vi "PictureParticleThreshold.vi"(5 "Enum":enum16{"new", "input", "draw", "dump"}(ring), 6 "spotfinding settings":T1={"show all"=FALSE, "threshold/morph"=FALSE, "particle filter"=FALSE, "spot marks"=FALSE, "close filter"=FALSE, "connectivity 4/8"=FALSE, "range"={"Lower value"=30.0, "Upper value"=30.0}, "PSF-size"=0, "Parameters"=[]} {"range"."Upper value" format="%.2f"; "range"."Lower value" format="%.2f"; "Parameters"."Upper Value" format="%.2f"; "Parameters"."Lower Value" format="%.2f"}, 8 "Image Input float":T2, 9 "Image Input 8bit":T2) -> (2 "Image Dst float":T2, 3 "Image Dst 8bit":T2)   [LabVIEW 2009]
uses:
  <vilib>/vision/Image Controls.llb/IMAQ Image.ctl
  spotfindersettings.ctl
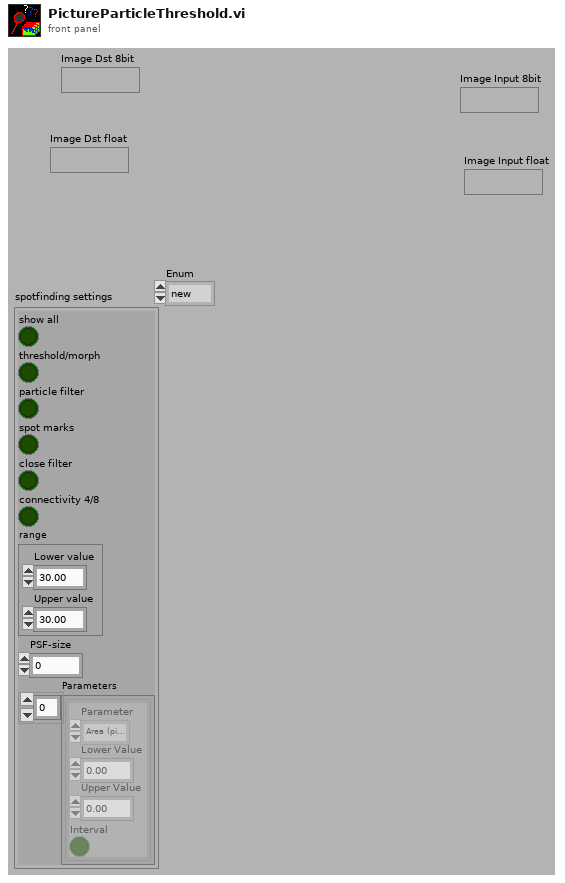
[diagram p1: front panel]
types:
  T1 = typedef "spotfindersettings.ctl" = cluster{"show all":bool, "threshold/morph":bool, "particle filter":bool, "spot marks":bool, "close filter":bool, "connectivity 4/8":bool, "range":cluster{"Lower value":sgl, "Upper value":sgl}, "PSF-size":i32, "Parameters":cluster{"Parameter":enum32{"Area (pixels)", "Area (calibrated)", "Number of holes", "Holes area (pixels)", "Total area (pixels)", "Scanned area (pixels)", "Ratio Area/Scanned area (%)", "Ratio Area/Total area (%)", "Center of mass (X)", "Center of mass (Y)", "Left column (X)", "Upper row (Y)", "Right column (X)", "Lower row (Y)", "Width (pixels)", "Height (pixels)", "Longest segment length", "Longest segment left column (X)", "Longest segment top row  (Y)", "Perimeter", "Holes perimeter", "SumX", "SumY", "SumXX", "SumYY", "SumXY", "Corrected projection X", "Corrected projection Y", "Moment of inertia Ixx", "Moment of inertia Iyy", "Moment of inertia Ixy", "Mean chord X", "Mean chord Y", "Max intercept", "Mean intercept perpendicular", "Particle orientation", "Equivalent ellipse minor axis", "Ellipse major axis", "Ellipse minor axis", "Ratio of equivalent ellipse axis", "Rectangle big side", "Rectangle small side", "Ratio of equivalent rectangle sides", "Elongation factor", "Compactness factor", "Heywood circularity factor", "Type factor", "Hydraulic radius", "Waddel disk diameter", "Diagonal"}, "Lower Value":sgl, "Upper Value":sgl, "Interval":bool}[]}
  T2 = typedef "IMAQ Image.ctl" = refnum<image>
  T3 = enum32{"Gray", "Binary", "Gradient", "Rainbow", "Temperature"}
  T4 = enum16{"Ini", "get", "dump", "set", "draw", "black"}
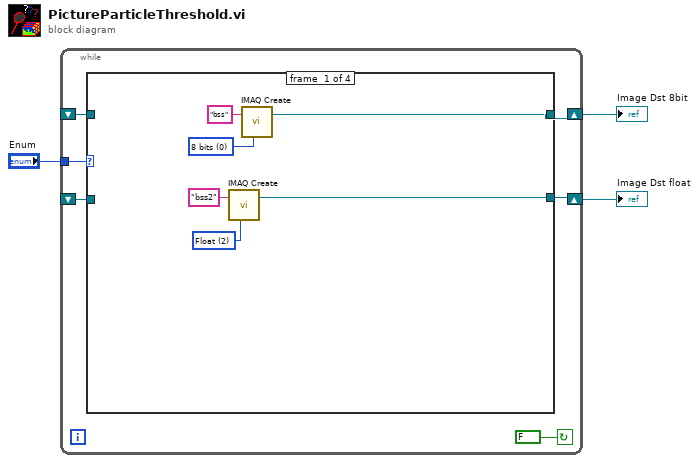
[diagram p0: block diagram]
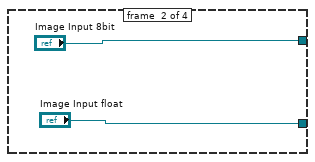
[diagram p2: hidden frame]
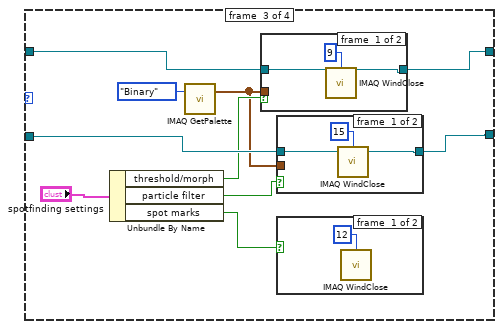
[diagram p3: hidden frame]
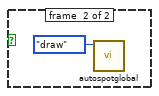
[diagram p4: hidden frame]
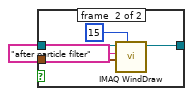
[diagram p5: hidden frame]
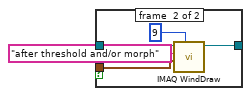
[diagram p6: hidden frame]
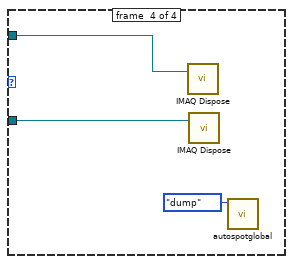
[diagram p7: hidden frame]
diagram:
  n1 = while {
    shift-right: [w9] -> w3
    shift-left: _ -> [w5]
    shift-right: [w8] -> w2
    shift-left: _ -> [w6]
    tunnel: "Enum" -> [w7]
    stop <- FALSE continue-if-true
    n2 = case shown="\"input\"" w7 {
      tunnel: [w11 "Image Input 8bit" w25 _] -> w9
      tunnel: [w10 "Image Input float" w27 _] -> w8
      tunnel: w6 -> [_ _ w26 w45]
      tunnel: w5 -> [_ _ w24 w46]
      frame #0 {
        w13 = u32 2 items=["8 bits", "16 bits", "Float", "Complex", "RGB", "HSL"] ("Image Type")
        w14 = u32 0 items=["8 bits", "16 bits", "Float", "Complex", "RGB", "HSL"] ("Image Type")
        n3 = call "IMAQ Create"("Image Name"="bss2", "Image Type"=w13) -> ("New Image"=w10:T2)  [unwired: 3 in, 1 out]
        n4 = call "IMAQ Create"("Image Name"="bss", "Image Type"=w14) -> ("New Image"=w11:T2)  [unwired: 3 in, 1 out]
      }
      frame #1 {
      }
      frame #2 {
        n5 = Unbundle By Name("spotfinding settings") -> ("threshold/morph"=w23:bool, "particle filter"=w22:bool, "spot marks"=w21:bool)
        n6 = call "IMAQ GetPalette"("Palette Number (gray)"=T3."Binary") -> ("Color Palette"=w19:cluster{"Red":u8, "Green":u8, "Blue":u8}[])  [unwired: 4 in, 1 out]
        n7 = case shown="False" w23 {
          tunnel: [w38 w41] -> w25
          tunnel: w24 -> [w38 w40]
          tunnel: w19 -> [_ w39]
          frame #0 {
            n8 = call "IMAQ WindClose"("Window Number (0...15)"=9) -> ()  [unwired: 5 in, 1 out]
          }
          frame #1 {
            n9 = call "IMAQ WindDraw"("Window Number (0...15)"=9, "Color Palette"=w39, "Title"="after threshold and/or morph", "Image"=w40) -> ("Image Out (duplicate)"=w41:T2)  [unwired: 6 in, 1 out]
          }
        }
        n10 = case shown="False" w22 {
          tunnel: [w31 w34] -> w27
          tunnel: w26 -> [w31 w33]
          tunnel: w19 -> [_ w32]
          frame #0 {
            n11 = call "IMAQ WindClose"("Window Number (0...15)"=15) -> ()  [unwired: 5 in, 1 out]
          }
          frame #1 {
            n12 = call "IMAQ WindDraw"("Window Number (0...15)"=15, "Color Palette"=w32, "Title"="after particle filter", "Image"=w33) -> ("Image Out (duplicate)"=w34:T2)  [unwired: 6 in, 1 out]
          }
        }
        n13 = case shown="False" w21 {
          frame #0 {
            n14 = call "IMAQ WindClose"("Window Number (0...15)"=12) -> ()  [unwired: 5 in, 1 out]
          }
          frame #1 {
            n15 = call "autospotglobal.vi"("Enum"=T4."draw") -> ()  [unwired: 6 in, 1 out]
          }
        }
      }
      frame #3 {
        n16 = call "IMAQ Dispose"("Image"=w46) -> ()  [unwired: 5 in, 1 out]
        n17 = call "IMAQ Dispose"("Image"=w45) -> ()  [unwired: 5 in, 1 out]
        n18 = call "autospotglobal.vi"("Enum"=T4."dump") -> ()  [unwired: 6 in, 1 out]
      }
    }
  }
  "Image Dst 8bit" <- w3
  "Image Dst float" <- w2
